vi "ATS_GetDriverVersion.vi"() -> (0 "Return Code":u32, 1 "Driver_#":u32 format="%09.0f", 2 "Driver_Version":string)   [LabVIEW 2010]
doc: "_____AlazarTech, Scope_____\n\nRetrieve the Driver version number.\n\nOutput:\n\"Driver_Version\" = version in text format.\n\"Dirver_#\" = version in U32 format.\n\nU32 format = (1st x 1E6) + (2nd x 1E3) + 3rd"
uses:
  ATSApi.dll
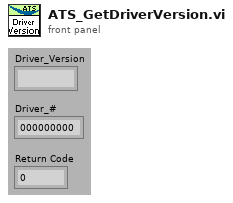
[diagram p1: front panel]
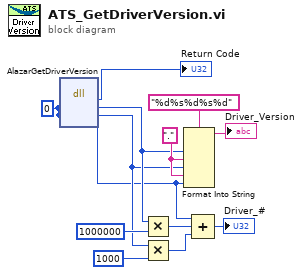
[diagram p0: block diagram]
diagram:
  w10 = u8 0
  w12 = "."
  n1 = dll-call lib="ATSApi.*" fn="AlazarGetDriverVersion"(w10, w10, w10) -> (→"Return Code":u32, w3:u8, w2:u8, w1:u8)  [unwired: 3 in, 2 out]
  n2 = Multiply(x=w3, y=u32 1000000) -> (x*y=w4:u32)
  n3 = Multiply(x=w2, y=u32 1000 ("x")) -> (x*y=w5:u32)
  n4 = Format Into String(format string="%d%s%d%s%d", w3, w12, w2, w12, w1) -> (resulting string=→"Driver_Version":string)  [unwired: 2 in, 1 out]
  n5 = Compound Arithmetic op=ADD(w1, w4, w5) -> (→"Driver_#":u32)
